vi "SVT Octave Spectrum Conversion (1 Ch).vi"(0 "octave spectrum":T6 {"band power" format="%.2f"; "nominal frequencies [Hz]" format="%.2f"}, 5 "desired scaling":T1 {"dB reference (0: no change)" format="%^_2e"}, 9 "octave info in":T2={"standard"=enum."ANSI S1.11", "bandwidth"=enum."1 octave", "low band"=0, "high band"=0, "weighting filter"=0, "dB reference"=0.0, "dB On"=FALSE, "unit label"="", "channel name"="", "description"="", "engineering units"=1, "custom label"="", "spectrum type"=enum."magnitude", "spectral density"=FALSE, "filters settled"=FALSE} {"engineering units" items=["custom..."=0, "V"=1, "A"=21, "C"=30, "pC"=31, "s"=32, "-"=29, "Pa"=2, "N"=20, "g"=3, "m/s^2"=4, "m/s"=5, "m"=6, "mm/s"=12, "mm"=13, "micron/s"=14, "micron"=15, "in/s^2"=7, "in/s"=8, "in"=9, "mil/s"=10, "mil"=11, "rad/s^2"=16, "rad/s"=17, "rad"=18, "deg/s^2"=26, "deg/s"=27, "deg"=28, "RPM"=22, "cycle/s^2"=23, "Hz"=24, "cycle"=25, "strain"=19]; "dB reference" format="%.2e"; "weighting filter" items=["Linear", "A-weighting", "B-weighting", "C-weighting", "ITU-R 468-4", "Dolby", "CCITT", "C-message", "Wb", "Wc", "Wd", "We", "Wf", "Wh", "Wj", "Wk", "Wm", "AES17 20 kHz lowpass", "AES17 40 kHz lowpass", "AES17 20 kHz highpass", "AES17 40 kHz highpass"]}, 11 "error in (no error)":errorcluster) -> (4 "converted octave spectrum":T6 {"band power" format="%.2f"; "nominal frequencies [Hz]" format="%.2f"}, 6 "unit label":string, 10 "octave info out":T2={"standard"=enum."ANSI S1.11", "bandwidth"=enum."1 octave", "low band"=0, "high band"=0, "weighting filter"=0, "dB reference"=0.0, "dB On"=FALSE, "unit label"="", "channel name"="", "description"="", "engineering units"=1, "custom label"="", "spectrum type"=enum."magnitude", "spectral density"=FALSE, "filters settled"=FALSE} {"engineering units" items=["custom..."=0, "V"=1, "A"=21, "C"=30, "pC"=31, "s"=32, "-"=29, "Pa"=2, "N"=20, "g"=3, "m/s^2"=4, "m/s"=5, "m"=6, "mm/s"=12, "mm"=13, "micron/s"=14, "micron"=15, "in/s^2"=7, "in/s"=8, "in"=9, "mil/s"=10, "mil"=11, "rad/s^2"=16, "rad/s"=17, "rad"=18, "deg/s^2"=26, "deg/s"=27, "deg"=28, "RPM"=22, "cycle/s^2"=23, "Hz"=24, "cycle"=25, "strain"=19]; "dB reference" format="%.2e"; "weighting filter" items=["Linear", "A-weighting", "B-weighting", "C-weighting", "ITU-R 468-4", "Dolby", "CCITT", "C-message", "Wb", "Wc", "Wd", "We", "Wf", "Wh", "Wj", "Wk", "Wm", "AES17 20 kHz lowpass", "AES17 40 kHz lowpass", "AES17 20 kHz highpass", "AES17 40 kHz highpass"]}, 15 "error out":errorcluster)   [LabVIEW 2017, in "SoundVib_Octave.lvlib"]
doc: "Converts an octave spectrum between dB/linear, magnitude/magnitude^2, spectrum/spectral density, and dB ref1/dB ref2. \n\nYou can use this VI to convert one octave spectrum or N octave spectra. Wire data to the <B>octave spectrum</B> input to determine the polymorphic instance to use or manually select the instance."
uses:
  <vilib>/addons/Sound and Vibration/svt_Octave/SoundVib_Octave.lvlib
  <vilib>/addons/_NISVFA/_Shared subVIs/Controls/svc_Octave Info.ctl
  <vilib>/addons/_NISVFA/_Shared subVIs/Controls/svc_Octave Standard.ctl
  <vilib>/addons/_NISVFA/_Shared subVIs/Controls/svc_Weighting Filter Text Ring.ctl
  <vilib>/addons/_NISVFA/_Shared subVIs/Controls/svc_Engineering Units Text Ring.ctl
  <vilib>/addons/Sound and Vibration/svt_Octave_2014 standard/SoundVib_Octave_2014 standard.lvlib
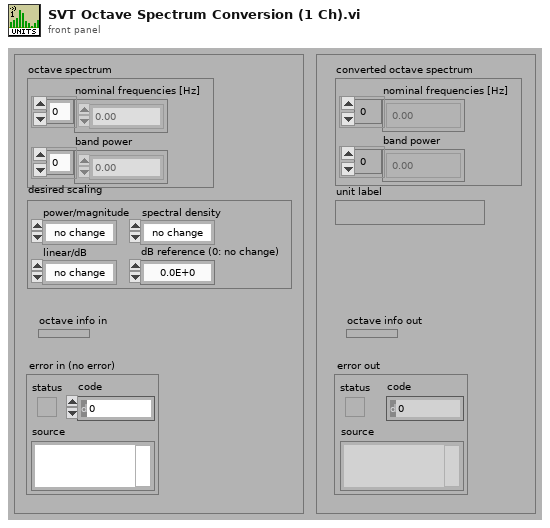
[diagram p1: front panel]
types:
  T1 = cluster{"linear/dB":enum16{"no change", "linear", "dB"}, "dB reference (0: no change)":dbl, "power/magnitude":enum16{"no change", "power", "magnitude"}, "spectral density":enum16{"no change", "spectrum", "spectral density"}}
  T2 = typedef "svc_Octave Info.ctl" = cluster{"standard":T3, "bandwidth":enum16{"1 octave", "1/3 octave", "1/6 octave", "1/12 octave", "1/24 octave"}, "low band":i32, "high band":i32, "weighting filter":T4, "dB reference":dbl, "dB On":bool, "unit label":string, "channel name":string, "description":string, "engineering units":T5, "custom label":string, "spectrum type":enum16{"power", "magnitude"}, "spectral density":bool, "filters settled":bool}
  T3 = typedef "svc_Octave Standard.ctl" = enum16{"ANSI S1.11", "IEC 61260"}
  T4 = typedef "svc_Weighting Filter Text Ring.ctl" = u16
  T5 = typedef "svc_Engineering Units Text Ring.ctl" = u16
  T6 = cluster{"nominal frequencies [Hz]":dbl[], "band power":dbl[]}
  T7 = enum16{"no change", "spectrum", "spectral density"}
  T8 = enum16{"1 octave", "1/3 octave", "1/6 octave", "1/12 octave", "1/24 octave", "1/48 octave", "1/96 octave"}
  T9 = enum16{"1 octave", "1/3 octave", "1/6 octave", "1/12 octave", "1/24 octave"}
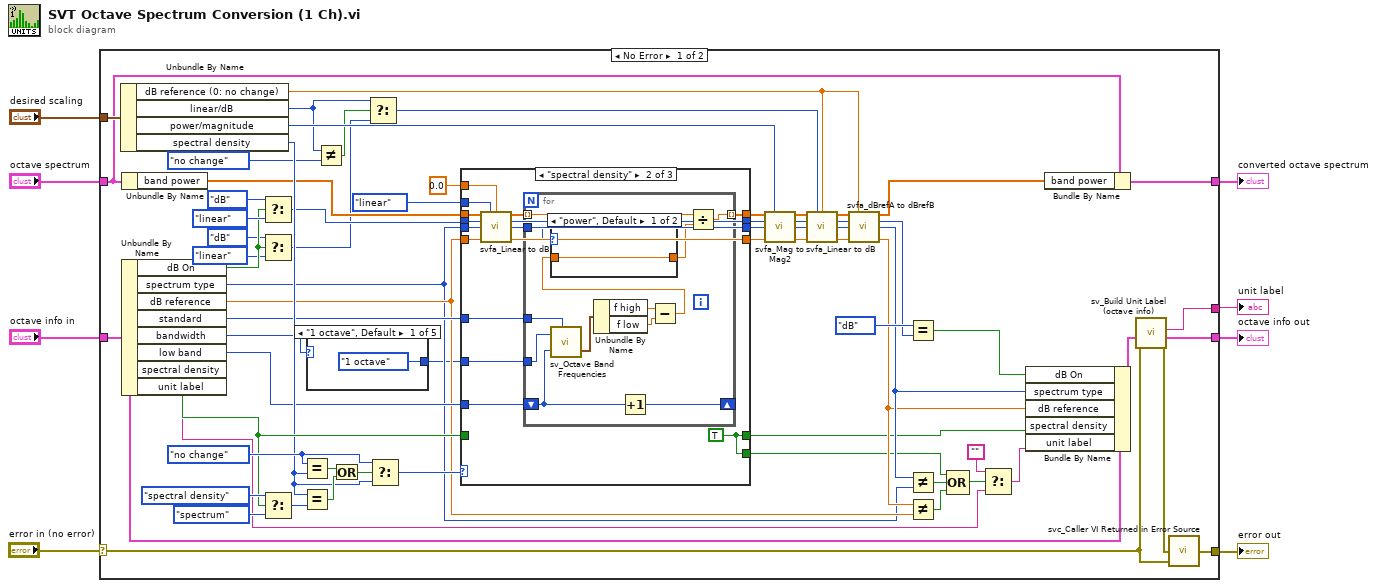
[diagram p0: block diagram]
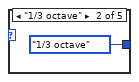
[diagram p2: hidden frame]
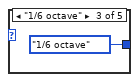
[diagram p3: hidden frame]
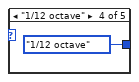
[diagram p4: hidden frame]
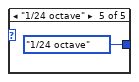
[diagram p5: hidden frame]
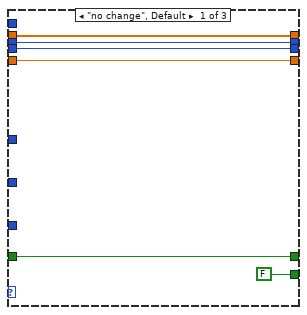
[diagram p6: hidden frame]
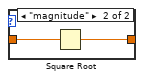
[diagram p7: hidden frame]
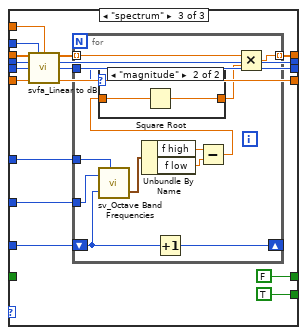
[diagram p8: hidden frame]
diagram:
  n1 = case shown="No Error" "error in (no error)" {
    selector: "error in (no error)" -> [w40 w150]
    tunnel: "octave spectrum" -> [w11 _]
    tunnel: "octave info in" -> [w64 w149]
    tunnel: [w75 w150] -> w8
    tunnel: [w39 _] -> w4
    tunnel: [w38 w149] -> w3
    tunnel: [w76 _] -> w2
    tunnel: "desired scaling" -> [w71 _]
    frame No Error {
      w54 = T7."no change" ("spectral density")
      n2 = Unbundle By Name(w71) -> ("dB reference (0: no change)"=w69:dbl, "linear/dB"=w14:enum16{"no change", "linear", "dB"}, "power/magnitude"=w35:enum16{"no change", "power", "magnitude"}, "spectral density"=w48:T7)
      n3 = Unbundle By Name(w11) -> ("band power"=w29:dbl[])
      n4 = Unbundle By Name(w64) -> ("dB On"=w17:bool, "spectrum type"=w19:enum16{"power", "magnitude"}, "dB reference"=w25:dbl, "standard"=w36:T3, "bandwidth"=w10:T9, "low band"=w47:i32, "spectral density"=w52:bool, "unit label"=w44:string)
      n5 = Select(t=enum16{"linear", "dB"}."dB" ("linear/dB"), s=w17, f=enum16{"linear", "dB"}."linear" ("linear/dB")) -> (s? t:f=w26:enum16{"linear", "dB"})
      n6 = Select(t=enum16{"no change", "linear", "dB"}."dB" ("y"), s=w17, f=enum16{"no change", "linear", "dB"}."linear" ("y")) -> (s? t:f=w12:enum16{"no change", "linear", "dB"})
      n7 = Select(t=T7."spectral density" ("spectral density"), s=w52, f=T7."spectrum" ("spectral density")) -> (s? t:f=w58:T7)
      n8 = Equal?(x=w54, y=w48) -> (x = y?=w57:bool)
      n9 = Equal?(x=w48, y=w58) -> (x = y?=w56:bool)
      n10 = case shown="\"1 octave\", Default" w10 {
        tunnel: [T8."1 octave" ("bandwidth") T8."1/3 octave" ("bandwidth") T8."1/6 octave" ("bandwidth") T8."1/12 octave" ("bandwidth") T8."1/24 octave" ("bandwidth")] -> w9
        frame "1 octave", Default {
        }
        frame "1/3 octave" {
        }
        frame "1/6 octave" {
        }
        frame "1/12 octave" {
        }
        frame "1/24 octave" {
        }
      }
      n11 = Not Equal?(x=w14, y=enum16{"no change", "linear", "dB"}."no change") -> (x != y?=w20:bool)
      n12 = Or(x=w57, y=w56) -> (x .or. y?=w55:bool)
      n13 = Select(t=w14, s=w20, f=w12) -> (s? t:f=w13:enum16{"no change", "linear", "dB"})
      n14 = Select(t=w54, s=w55, f=w48) -> (s? t:f=w53:T7)
      n15 = case shown="\"spectral density\"" w53 {
        tunnel: [w87 w102 w133] -> w34
        tunnel: w29 -> [w87 w98 w128]
        tunnel: w52 -> [w86 _ _]
        tunnel: [w86 w100 FALSE ("spectral density")] -> w51
        tunnel: w47 -> [_ w101 w132]
        tunnel: [FALSE ("spectral density") w100 TRUE ("spectral density")] -> w46
        tunnel: w36 -> [_ w99 w129]
        tunnel: 0.0 ("dB reference (desired)") -> [_ w96 w125]
        tunnel: enum16{"no change", "linear", "dB"}."linear" ("linear/dB desired") -> [_ w95 w126]
        tunnel: w26 -> [w84 w94 w124]
        tunnel: w19 -> [w83 w93 w123]
        tunnel: w25 -> [w82 w92 w122]
        tunnel: [w84 w91 w121] -> w24
        tunnel: [w83 w89 w119] -> w23
        tunnel: [w82 w90 w120] -> w22
        tunnel: w9 -> [_ w88 w118]
        frame "no change", Default {
        }
        frame "spectral density" {
          w100 = TRUE ("spectral density")
          n16 = call <vilib>:"svfa_Linear to dB.vi"("input signal"=w98, "linear/dB desired"=w95, "dB reference (desired)"=w96, "linear/dB (in)"=w94, "power/magnitude"=w93, "dB reference"=w92) -> ("converted signal"=w97:dbl[], "linear/dB (out)"=w91:enum16{"linear", "dB"}, "power/magnitude (dupl)"=w89:enum16{"power", "magnitude"}, "dB reference (dupl)"=w90:dbl)  [unwired: 5 in, 1 out]
          n17 = for {
            tunnel: w97 -> [w109] mode=indexing
            shift-right: [w114] -> _
            shift-left: w101 -> [w113]
            tunnel: [w108] -> w102 mode=indexing
            tunnel: w99 -> [w107]
            tunnel: w89 -> [w106]
            tunnel: w88 -> [w103]
            n18 = call <vilib>:"sv_Octave Band Frequencies.vi"("octave band selector"=w113, "bandwidth"=w103, "standard"=w107) -> ("bandedge frequencies [Hz]"=w112:cluster{"f low":dbl, "f high":dbl})  [unwired: 1 in, 3 out]
            n19 = Unbundle By Name(w112) -> ("f high"=w111:dbl, "f low"=w110:dbl)
            n20 = Increment(x=w113) -> (x+1=w114:i32)
            n21 = Subtract(x=w111, y=w110) -> (x-y=w105:dbl)
            n22 = case shown="\"power\", Default" w106 {
              tunnel: w105 -> [w115 w117]
              tunnel: [w115 w116] -> w104
              frame "power", Default {
              }
              frame "magnitude" {
                n23 = Square Root(x=w117) -> (sqrt(x)=w116:dbl)
              }
            }
            n24 = Divide(x=w109, y=w104) -> (x/y=w108:dbl)
          }
        }
        frame "spectrum" {
          n25 = call <vilib>:"svfa_Linear to dB.vi"("input signal"=w128, "linear/dB desired"=w126, "dB reference (desired)"=w125, "linear/dB (in)"=w124, "power/magnitude"=w123, "dB reference"=w122) -> ("converted signal"=w127:dbl[], "linear/dB (out)"=w121:enum16{"linear", "dB"}, "power/magnitude (dupl)"=w119:enum16{"power", "magnitude"}, "dB reference (dupl)"=w120:dbl)  [unwired: 5 in, 1 out]
          n26 = for {
            tunnel: w127 -> [w140] mode=indexing
            shift-right: [w145] -> _
            shift-left: w132 -> [w144]
            tunnel: [w139] -> w133 mode=indexing
            tunnel: w129 -> [w138]
            tunnel: w119 -> [w137]
            tunnel: w118 -> [w134]
            n27 = call <vilib>:"sv_Octave Band Frequencies.vi"("octave band selector"=w144, "bandwidth"=w134, "standard"=w138) -> ("bandedge frequencies [Hz]"=w143:cluster{"f low":dbl, "f high":dbl})  [unwired: 1 in, 3 out]
            n28 = Unbundle By Name(w143) -> ("f high"=w142:dbl, "f low"=w141:dbl)
            n29 = Increment(x=w144) -> (x+1=w145:i32)
            n30 = Subtract(x=w142, y=w141) -> (x-y=w136:dbl)
            n31 = case shown="\"magnitude\"" w137 {
              tunnel: w136 -> [w146 w148]
              tunnel: [w146 w147] -> w135
              frame "power", Default {
              }
              frame "magnitude" {
                n32 = Square Root(x=w148) -> (sqrt(x)=w147:dbl)
              }
            }
            n33 = Multiply(x=w140, y=w135) -> (x*y=w139:dbl)
          }
        }
      }
      n34 = call <vilib>:"svfa_Mag to Mag2.vi"("input signal"=w34, "power/magnitude desired"=w35, "linear/dB"=w24, "power/magnitude"=w23, "dB reference"=w22) -> ("converted signal"=w33:dbl[], "dup linear/dB"=w32:enum16{"linear", "dB"}, "power/magnitude (out)"=w31:enum16{"power", "magnitude"}, "dB reference (out)"=w30:dbl)  [unwired: 6 in, 1 out]
      n35 = call <vilib>:"svfa_Linear to dB.vi"("input signal"=w33, "linear/dB desired"=w13, "dB reference (desired)"=w69, "linear/dB (in)"=w32, "power/magnitude"=w31, "dB reference"=w30) -> ("converted signal"=w74:dbl[], "linear/dB (out)"=w68:enum16{"linear", "dB"}, "power/magnitude (dupl)"=w67:enum16{"power", "magnitude"}, "dB reference (dupl)"=w70:dbl)  [unwired: 5 in, 1 out]
      n36 = call <vilib>:"svfa_dBrefA to dBrefB.vi"("input signal"=w74, "dB reference (desired)"=w69, "linear/dB"=w68, "power/magnitude"=w67, "dB reference"=w70) -> ("converted signal"=w73:dbl[], "linear/dB (dupl)"=w65:enum16{"linear", "dB"}, "power/magnitude (dupl)"=w63:enum16{"power", "magnitude"}, "dB reference (out)"=w61:dbl)  [unwired: 6 in, 1 out]
      n37 = Equal?(x=enum16{"linear", "dB"}."dB" ("linear/dB"), y=w65) -> (x = y?=w62:bool)
      n38 = Not Equal?(x=w63, y=w19) -> (x != y?=w49:bool)
      n39 = Not Equal?(x=w61, y=w25) -> (x != y?=w50:bool)
      n40 = Compound Arithmetic op=OR(w46, w49, w50) -> (w45:bool)
      n41 = Select(t="", s=w45, f=w44) -> (s? t:f=w42:string)
      n42 = Bundle By Name(cluster=w64, "dB On"=w62, "spectrum type"=w63, "dB reference"=w61, "spectral density"=w51, "unit label"=w42) -> (w41:T2)
      n43 = Bundle By Name(cluster=w11, "band power"=w73) -> (w76:T6)
      n44 = call <vilib>:"sv_Build Unit Label (octave info).vi"("error in (no error)"=w40, "octave info"=w41) -> ("error out"=w37:errorcluster, "octave info out"=w38:T2, "unit label"=w39:string)  [unwired: 7 in]
      n45 = call <vilib>:"svc_Caller VI Returned in Error Source.vi"("warning input to caller"=w40, "error in (no error)"=w37) -> ("error out"=w75:errorcluster)  [unwired: 3 in]
    }
    frame Error {
    }
  }
  "error out" <- w8
  "converted octave spectrum" <- w2
  "octave info out" <- w3
  "unit label" <- w4
